vi "SeuilAuto.vi"(11 "V target":refnum<vi>) -> (1 "Seuil V":dbl, 2 "Largeur P":dbl, 3 "Seuil P":dbl, 4 "Largeur V":dbl)   [LabVIEW 2023]
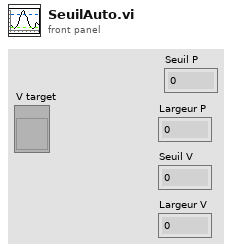
[diagram p1: front panel]
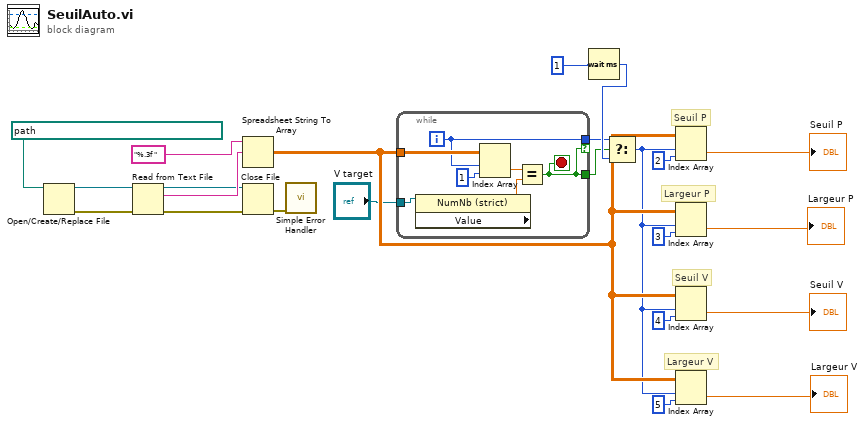
[diagram p0: block diagram]
diagram:
  # "Largeur V"
  # "Largeur P"
  # "Seuil V"
  # "Seuil P"
  n1 = Open/Create/Replace File(file path (use dialog)=path "D:/Documents/Mémoire/Data John Doe/Fichiers excels/Config Seuil-Largeur_P-V(tab).txt" ("chemin du fichier (utiliser une boîte de dialogue)")) -> (refnum out=w16:refnum<file>, error out=w15:errorcluster)  [unwired: 5 in, 1 out]
  n2 = Read from Text File(file (use dialog)=w16, error in=w15) -> (refnum out=w17:refnum<file>, text=w19:string, error out=w18:errorcluster)  [unwired: 2 in, 1 out]
  n3 = Spreadsheet String To Array(format string="%.3f ", spreadsheet string=w19) -> (array=w23:dbl[][])  [unwired: 2 in]
  n4 = Close File(refnum=w17, error in=w18) -> (error out=w21:errorcluster)  [unwired: 1 out]
  n5 = call <vilib>:"Simple Error Handler.vi"("error in (no error)"=w21) -> ()  [unwired: 4 in, 5 out]
  n6 = while {
    tunnel: w23 -> [w29]
    tunnel: [w27] -> w7 if=w26
    tunnel: [w26] -> w6
    tunnel: "V target" -> [w24]
    i -> [w27]
    stop <- w26 stop-if-true
    n7 = property class="NumNb (strict)"(reference=w24) -> ("Value"=w25:dbl)  [unwired: 1 in, 2 out]
    n8 = Index Array(array=w29, index (row)=w27, index (col)=1 ("indice (col)")) -> (element=w28:dbl)
    n9 = Equal?(x=w28, y=w25) -> (x = y?=w26:bool)
  }
  n10 = Wait (ms)(milliseconds to wait=u32 1 ("attente (ms)")) -> (millisecond timer value=w9:u32)
  n11 = Select(t=w7, s=w6, f=w9) -> (s? t:f=w8:u32)
  n12 = Index Array(array=w23, index (row)=w8, index (col)=2 ("indice (col)")) -> (element=→"Seuil P":dbl)
  n13 = Index Array(array=w23, index (row)=w8, index (col)=3 ("indice (col)")) -> (element=→"Largeur P":dbl)
  n14 = Index Array(array=w23, index (row)=w8, index (col)=4 ("indice (col)")) -> (element=→"Seuil V":dbl)
  n15 = Index Array(array=w23, index (row)=w8, index (col)=5 ("indice (col)")) -> (element=→"Largeur V":dbl)
